vi "globals0.vi"() -> ()   [LabVIEW 2011]
panel:
  out "Growth Sequence Preferences":path=path "C:/MOCVD/GrowthSequencePreferences.ini"
  out "Growth Database":path=path "C:/MOCVD/MOCVD_Growths.accdb"
  out "Log Path":path
  out "Last Step":i32
  out "Seq Step Time (s)":dbl=0.01
  out "Current Time":timestamp
  out "Begin Time":timestamp
  out "Temperature Controller RS232":refnum<visa-resource-name>="COM1"
  out "Log String":string
  out "Byte Stream File Refnum":refnum<file>
  out "Log File Path":path
  out "GPIB Address":string="23"
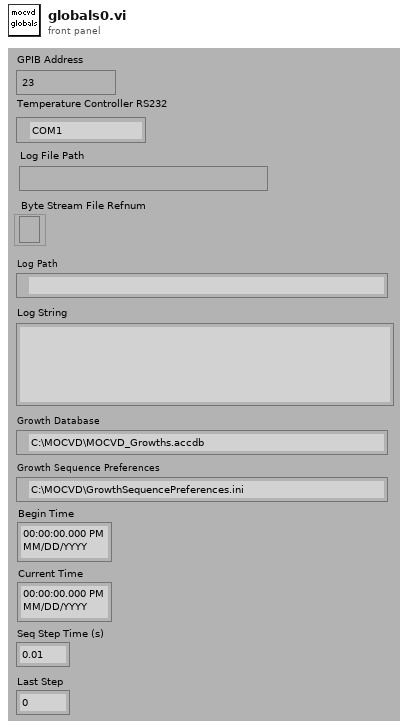
[diagram p1: front panel]
diagram:
